vi "ClimbExecute.vi"   [LabVIEW 2023]
uses:
  <vilib>/Rock Robotics/WPI/ThirdParty/JAS_Junk/TrajLib/Trajectory_Library.lvlib
  <vilib>/Rock Robotics/Network Tables/NT Write Number.vi
  <vilib>/Rock Robotics/Network Tables/NT Write Boolean.vi
types:
  T1 = typedef "WPI_MotorControlDeviceRef.ctl" = cluster{"DeviceStatus":errorcluster, "Type":T2, "PWM":cluster{"PWM Channel":T3, "DeadBand":T4}, "CAN":cluster{"Device Number":u8, "SetOutput VI Ref":variant, "GetOutput VI Ref":variant, "Enable VI Ref":variant, "Disable VI Ref":variant, "Data":variant}, "Invert":bool, "DIO PWM":cluster{"PWM \"Enable\" Channel":T3, "DIOChannel":T5, "PWM Rate":dbl}}
  T2 = typedef "WPI_MotorControlType.ctl" = enum16{"PWM", "CAN", "DIO PWM"}
  T3 = typedef "FPGA_DIOPWMChannel.ctl" = enum8{"PWM 0", "PWM 1", "PWM 2", "PWM 3", "PWM 4", "PWM 5", "PWM 6", "PWM 7", "PWM 8", "PWM 9", "PWM MXP 0", "PWM MXP 1", "PWM MXP 2", "PWM MXP 3", "PWM MXP 4", "PWM MXP 5", "PWM MXP 6", "PWM MXP 7", "PWM MXP 8", "PWM MXP 9", "Invalid"}
  T4 = typedef "WPI_PWMDeadband.ctl" = cluster{"Name":string, "maxPositivePwm":i32, "minPositivePwm":i32, "centerPwm":i32, "maxNegativePwm":i32, "minNegativePwm":i32, "angularRange":u16}
  T5 = typedef "FPGA_DIOChannel.ctl" = enum8{"DIO 0", "DIO 1", "DIO 2", "DIO 3", "DIO 4", "DIO 5", "DIO 6", "DIO 7", "DIO 8", "DIO 9", "DIO MXP 0", "DIO MXP 1", "DIO MXP 2", "DIO MXP 3", "DIO MXP 4", "DIO MXP 5", "DIO MXP 6", "DIO MXP 7", "DIO MXP 8", "DIO MXP 9", "DIO MXP 10", "DIO MXP 11", "DIO MXP 12", "DIO MXP 13", "DIO MXP 14", "DIO MXP 15", "SPI Port CS1", "SPI Port CS2", "SPI Port CS3", "SPI Port MISO", "SPI Port MOSI", "Invalid"}
  T6 = typedef "Trajectory_Library.lvlib/PosCtrl_Tuning_Type.ctl" = cluster{"Slope":dbl, "Offset":dbl, "Error Deadband":dbl, "At Reference Count":i32, "Negate Output":bool, "Max Allowd Position":dbl, "Min Allowd Position":dbl}
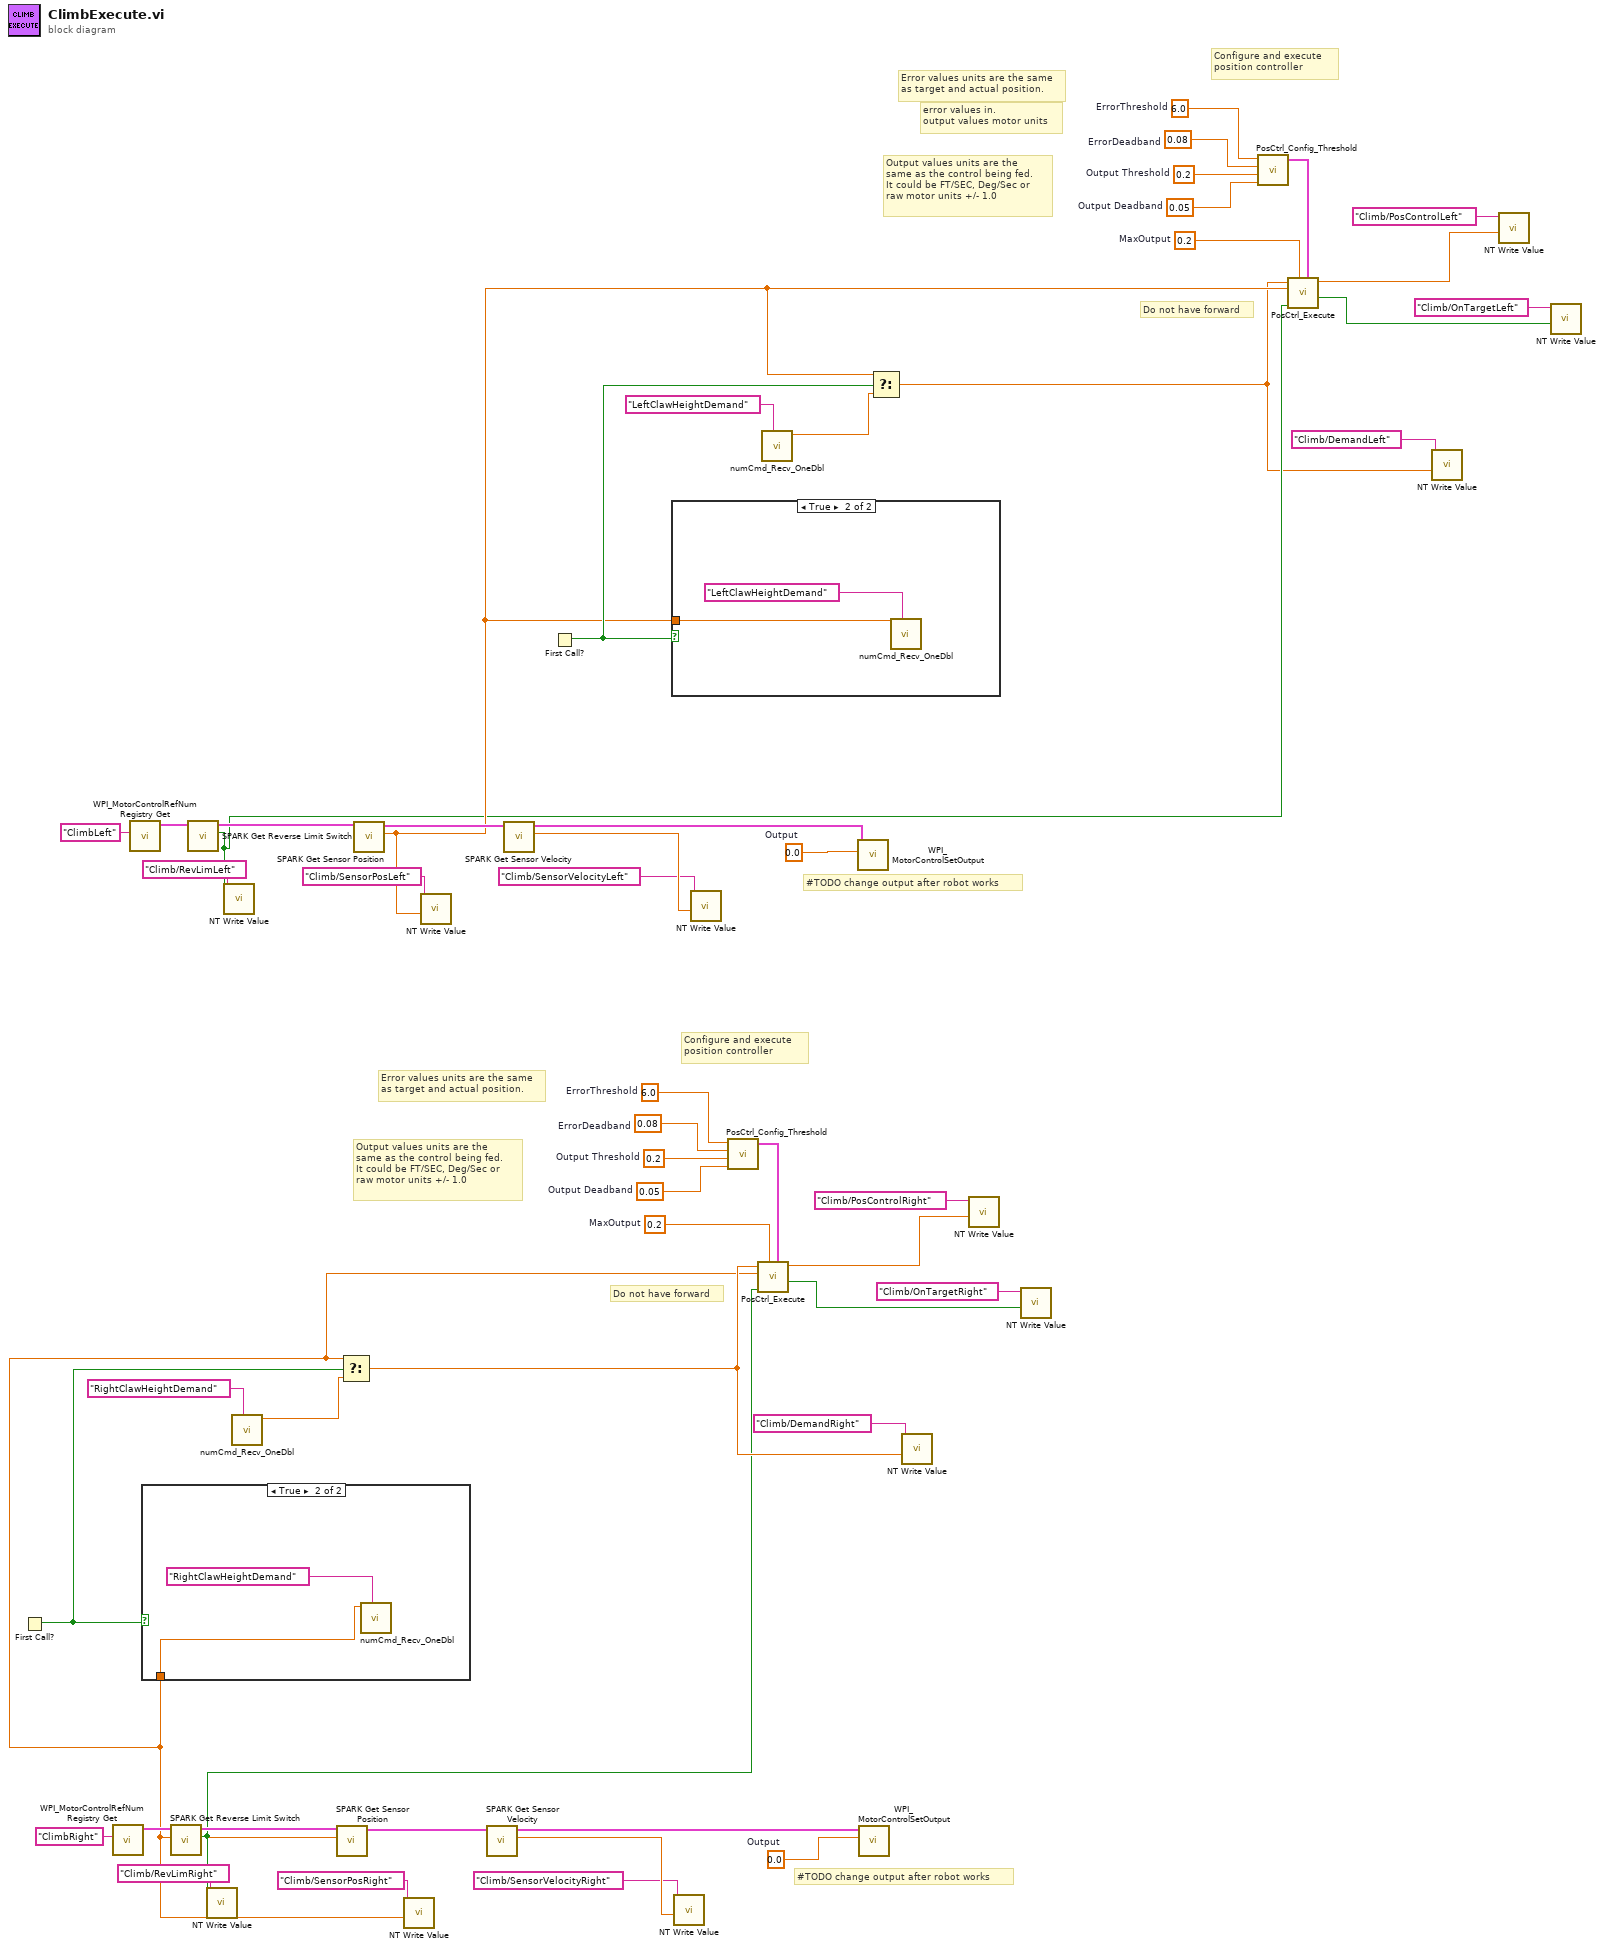
[diagram p0: block diagram]
diagram:
  w2 = 0.0  # Output
  w19 = 0.2  # MaxOutput
  w17 = 6.0  # ErrorThreshold
  w16 = 0.08  # ErrorDeadband
  w15 = 0.2  # Output Threshold
  w14 = 0.05  # Output Deadband
  w26 = 0.0  # Output
  w54 = 0.2  # MaxOutput
  w52 = 6.0  # ErrorThreshold
  w51 = 0.08  # ErrorDeadband
  w50 = 0.2  # Output Threshold
  w49 = 0.05  # Output Deadband
  # "error values in.\noutput values motor units"
  # "#TODO change output after robot works"
  # "Do not have forward"
  # "Output values units are the\nsame as the control being fed.  \nIt could be FT/SEC, Deg/Sec or\nraw motor units +/- 1.0"
  # "Error values units are the same \nas target and actual position."
  # "Configure and execute \nposition controller"
  # "#TODO change output after robot works"
  # "Do not have forward"
  # "Output values units are the\nsame as the control being fed.  \nIt could be FT/SEC, Deg/Sec or\nraw motor units +/- 1.0"
  # "Error values units are the same \nas target and actual position."
  # "Configure and execute \nposition controller"
  n1 = First Call?() -> (First Call?: T/F=w13:bool)
  n2 = call <vilib>:"WPI_MotorControlRefNum Registry Get.vi"("refnum name"="ClimbRight") -> ("MotorControlDevRef"=w40:T1)  [unwired: 9 in, 1 out]
  n3 = call <vilib>:"WPI_MotorControlRefNum Registry Get.vi"("refnum name"="ClimbLeft") -> ("MotorControlDevRef"=w48:T1)  [unwired: 9 in, 1 out]
  n4 = call <vilib>:"SPARK Get Reverse Limit Switch.vi"("MotorControlDevRef in"=w40) -> ("Hard Limit Rev"=w5:bool, "MotorControlDevRef out"=w37:T1)  [unwired: 7 in, 2 out]
  n5 = call <vilib>:"SPARK Get Reverse Limit Switch.vi"("MotorControlDevRef in"=w48) -> ("Hard Limit Rev"=w28:bool, "MotorControlDevRef out"=w45:T1)  [unwired: 7 in, 2 out]
  n6 = call-poly <vilib>:"NT Write Value.vi"("value"=w5, "name"="Climb/RevLimRight") -> ()  [unwired: 9 in, 1 out]
  n7 = call-poly <vilib>:"NT Write Value.vi"("value"=w28, "name"="Climb/RevLimLeft") -> ()  [unwired: 9 in, 1 out]
  n8 = call <vilib>:"numCmd_Recv_OneDbl.vi"("Command Name"="RightClawHeightDemand") -> ("Value"=w11:dbl)  [unwired: 8 in, 2 out]
  n9 = call <vilib>:"SPARK Get Sensor Position.vi"("MotorControlDevRef in"=w37) -> ("Sensor Position"=w4:dbl, "MotorControlDevRef out"=w39:T1)  [unwired: 7 in, 2 out]
  n10 = case shown="True" w13 {
    tunnel: w4 -> [_ w55]
    frame False {
    }
    frame True {
      n11 = call <vilib>:"numCmd_Recv_OneDbl.vi"("Command Name"="RightClawHeightDemand", "Initial Value"=w55) -> ()  [unwired: 7 in, 3 out]
    }
  }
  n12 = Select(t=w4, s=w13, f=w11) -> (s? t:f=w10:dbl)
  n13 = call <vilib>:"SPARK Get Sensor Position.vi"("MotorControlDevRef in"=w45) -> ("Sensor Position"=w31:dbl, "MotorControlDevRef out"=w47:T1)  [unwired: 7 in, 2 out]
  n14 = call-poly <vilib>:"NT Write Value.vi"("value"=w4, "name"="Climb/SensorPosRight") -> ()  [unwired: 9 in, 1 out]
  n15 = call-poly <vilib>:"NT Write Value.vi"("value"=w31, "name"="Climb/SensorPosLeft") -> ()  [unwired: 9 in, 1 out]
  n16 = call <vilib>:"SPARK Get Sensor Velocity.vi"("MotorControlDevRef in"=w39) -> ("Sensor Velocity"=w34:dbl, "MotorControlDevRef out"=w1:T1)  [unwired: 7 in, 2 out]
  n17 = call <vilib>:"SPARK Get Sensor Velocity.vi"("MotorControlDevRef in"=w47) -> ("Sensor Velocity"=w42:dbl, "MotorControlDevRef out"=w27:T1)  [unwired: 7 in, 2 out]
  n18 = First Call?() -> (First Call?: T/F=w32:bool)
  n19 = case shown="True" w32 {
    tunnel: w31 -> [_ w57]
    frame False {
    }
    frame True {
      n20 = call <vilib>:"numCmd_Recv_OneDbl.vi"("Command Name"="LeftClawHeightDemand", "Initial Value"=w57) -> ()  [unwired: 7 in, 3 out]
    }
  }
  n21 = call-poly <vilib>:"NT Write Value.vi"("value"=w34, "name"="Climb/SensorVelocityRight") -> ()  [unwired: 9 in, 1 out]
  n22 = call-poly <vilib>:"NT Write Value.vi"("value"=w42, "name"="Climb/SensorVelocityLeft") -> ()  [unwired: 9 in, 1 out]
  n23 = call <vilib>:"PosCtrl_Config_Threshold.vi"("Output Deadband"=w14, "Output Threshold"=w15, "ErrorDeadband"=w16, "ErrorThreshold"=w17) -> ("PosCtrl_Config_Params"=w18:T6)  [unwired: 7 in]
  n24 = call <vilib>:"PosCtrl_Execute.vi"("PosCtrl_Config_Params"=w18, "MaxOutput"=w19, "Rev Limit Switch"=w5, "CurrentPosition"=w4, "TargetPosition"=w10) -> ("OnTarget"=w7:bool, "Output"=w8:dbl)  [unwired: 4 in, 1 out]
  n25 = call <vilib>:"numCmd_Recv_OneDbl.vi"("Command Name"="LeftClawHeightDemand") -> ("Value"=w29:dbl)  [unwired: 8 in, 2 out]
  n26 = call <vilib>:"WPI_MotorControlSetOutput.vi"("Output"=w26, "MotorControlDevRef"=w27) -> ()  [unwired: 7 in, 3 out]
  n27 = call <vilib>:"WPI_MotorControlSetOutput.vi"("Output"=w2, "MotorControlDevRef"=w1) -> ()  [unwired: 7 in, 3 out]
  n28 = Select(t=w31, s=w32, f=w29) -> (s? t:f=w25:dbl)
  n29 = call-poly <vilib>:"NT Write Value.vi"("value"=w10, "name"="Climb/DemandRight") -> ()  [unwired: 9 in, 1 out]
  n30 = call-poly <vilib>:"NT Write Value.vi"("value"=w8, "name"="Climb/PosControlRight") -> ()  [unwired: 9 in, 1 out]
  n31 = call-poly <vilib>:"NT Write Value.vi"("value"=w7, "name"="Climb/OnTargetRight") -> ()  [unwired: 9 in, 1 out]
  n32 = call <vilib>:"PosCtrl_Config_Threshold.vi"("Output Deadband"=w49, "Output Threshold"=w50, "ErrorDeadband"=w51, "ErrorThreshold"=w52) -> ("PosCtrl_Config_Params"=w53:T6)  [unwired: 7 in]
  n33 = call <vilib>:"PosCtrl_Execute.vi"("PosCtrl_Config_Params"=w53, "MaxOutput"=w54, "Rev Limit Switch"=w28, "CurrentPosition"=w31, "TargetPosition"=w25) -> ("OnTarget"=w21:bool, "Output"=w23:dbl)  [unwired: 4 in, 1 out]
  n34 = call-poly <vilib>:"NT Write Value.vi"("value"=w25, "name"="Climb/DemandLeft") -> ()  [unwired: 9 in, 1 out]
  n35 = call-poly <vilib>:"NT Write Value.vi"("value"=w23, "name"="Climb/PosControlLeft") -> ()  [unwired: 9 in, 1 out]
  n36 = call-poly <vilib>:"NT Write Value.vi"("value"=w21, "name"="Climb/OnTargetLeft") -> ()  [unwired: 9 in, 1 out]
